vi "WriteI32Data.vi"(8 "Error In":errorcluster caption="エラー入力", 9 "数値":i32, 10 "データ":T2, 11 "refnum":T1) -> (0 "Error Out":errorcluster caption="エラー出力", 3 "refnum out":T1 caption="refnum出力")   [LabVIEW 2015]
doc: "iniファイルからI32データを読み込みます。"
uses:
  <vilib>/Utility/config.llb/Config Data RefNum.ctl
  <vilib>/Utility/config.llb/Write Key (I32).vi
  <vilib>/Utility/config.llb/NI_LVConfig.lvlib
panel:
  # "■IniファイルへI32データを書き込む"
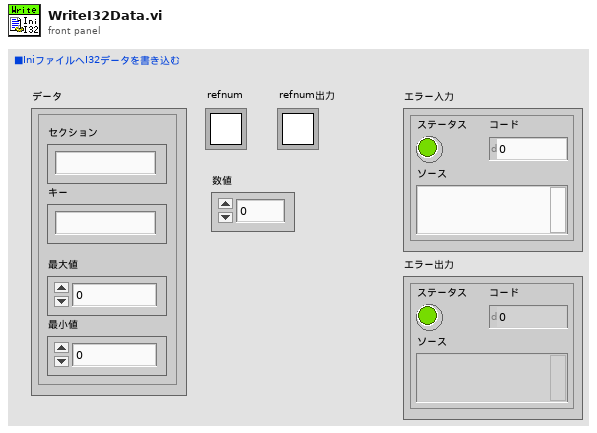
[diagram p1: front panel]
types:
  T1 = typedef "NI_LVConfig.lvlib/Config Data RefNum.ctl" = refnum<k1>
  T2 = cluster{"セクション":string, "キー":string, "最大値":i32, "最小値":i32}
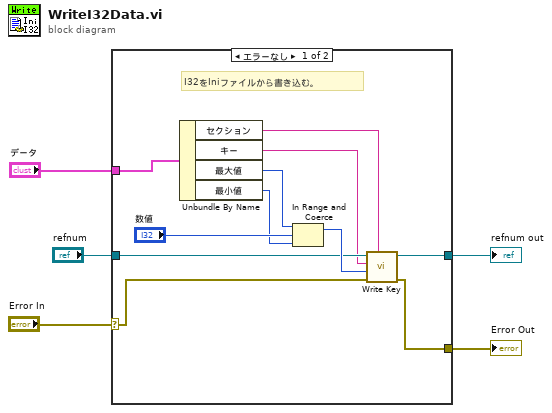
[diagram p0: block diagram]
diagram:
  n1 = case shown="エラーなし" "Error In" {
    selector: "Error In" -> [w7 w18]
    tunnel: [w6 w18] -> w5
    tunnel: "データ" -> [w16 _]
    tunnel: [w8 w17] -> w2
    tunnel: "refnum" -> [w11 w17]
    frame No Error {
      # "I32をIniファイルから書き込む。"
      n2 = Unbundle By Name(w16) -> ("セクション"=w10:string, "キー"=w9:string, "最大値"=w14:i32, "最小値"=w13:i32)
      n3 = In Range and Coerce(upper limit=w14, x="数値", lower limit=w13) -> (coerced(x)=w12:i32)  [unwired: 1 out]
      n4 = call-poly <vilib>:"Write Key.vi"("section"=w10, "error in (no error)"=w7, "value"=w12, "key"=w9, "refnum"=w11) -> ("error out"=w6:errorcluster, "refnum out"=w8:T1)  [unwired: 4 in, 1 out]
    }
    frame Error {
    }
  }
  "Error Out" <- w5
  "refnum out" <- w2
